vi "Add to Statistics.vi"(10 "Non Object":refnum<class "JSON Value.lvclass">, 11 "JSON Value In":refnum<class "JSON Value.lvclass">) -> (3 "JSON Statistics out":refnum<class "JSON Statistics.lvclass">)   [LabVIEW 2020, in "Library Commun.lvlib" / "JSON Value.lvclass"]
uses:
  JSON Value.lvclass
  Statistics/JSON Statistics.lvclass
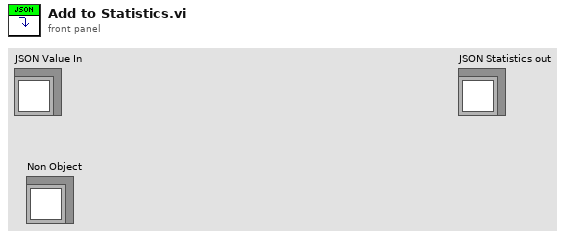
[diagram p1: front panel]
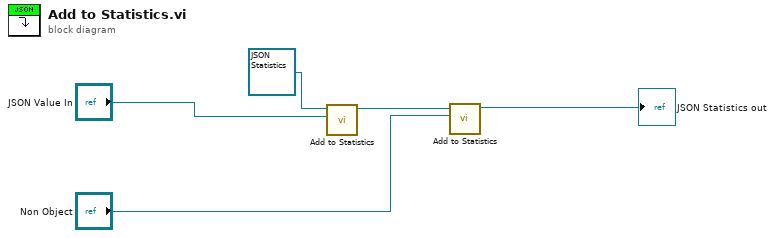
[diagram p0: block diagram]
diagram:
  n1 = call-dynamic "Add to Statistics.vi"("Non Object"="JSON Value In", "JSON Statistics in"=refnum<class "JSON Statistics.lvclass"> refnum) -> ("JSON Statistics out"=w3:refnum<class "JSON Statistics.lvclass">)  [unwired: 9 in]
  n2 = call-dynamic "Add to Statistics.vi"("Non Object"="Non Object", "JSON Statistics in"=w3) -> ("JSON Statistics out"=→"JSON Statistics out":refnum<class "JSON Statistics.lvclass">)  [unwired: 9 in]
